vi "Bipolar Output (Read).vi"(6 "ISOBUS address":T2=-1 caption="ISOBUS address (-1)", 8 "error in":errorcluster, 11 "Mercury Reference In":T3) -> (0 "error out":errorcluster, 2 "Bipolar Output":string, 3 "Mercury Reference Out":T3, 4 "Valid?":T1)   [LabVIEW 2013, in "Mercury iXX.lvlib" / "Magnet.lvlib"]
doc: "Read the Bipolar output mode of the selected magnet PSU."
uses:
  <instrlib>/Mercury iXX/Public/Libraries/Magnet.lvlib
  <instrlib>/Mercury iXX/Public/Controls/Mercury Reference.ctl
  <instrlib>/Mercury iXX/Public/Controls/Comms Transport Layer.ctl
  <instrlib>/Mercury iXX/Private/Controls/Query Dynamic Reference.ctl
  <instrlib>/Mercury iXX/Public/Controls/ISOBus Address.ctl
  <instrlib>/Mercury iXX/Public/Controls/Is Valid LED.ctl
  <instrlib>/Mercury iXX/Private/Controls/Command Verbs.ctl
  <instrlib>/Mercury iXX/Mercury iXX.lvlib
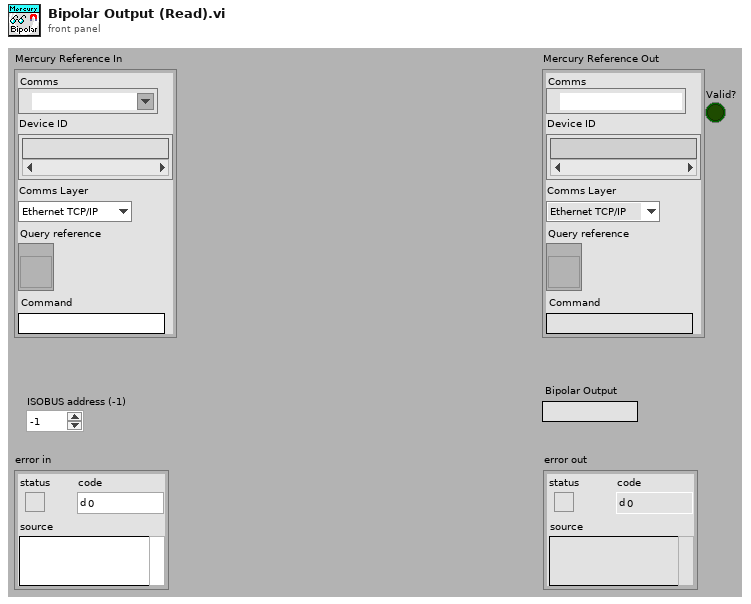
[diagram p1: front panel]
types:
  T1 = typedef "Mercury iXX.lvlib/Is Valid LED.ctl" = bool
  T2 = typedef "Mercury iXX.lvlib/ISOBus Address.ctl" = i32
  T3 = typedef "Mercury iXX.lvlib/Mercury Reference.ctl" = cluster{"Comms":refnum<visa-resource-name>, "Device ID":string[], "Comms Layer":T4, "Command":string, "Query reference":T5}
  T4 = typedef "Mercury iXX.lvlib/Comms Transport Layer.ctl" = enum16{"Ethernet TCP/IP", "USB", "ISOBus - RS-232", "GPIB"}
  T5 = typedef "Mercury iXX.lvlib/Query Dynamic Reference.ctl" = refnum<vi>
  T6 = typedef "Mercury iXX.lvlib/Command Verbs.ctl" = string
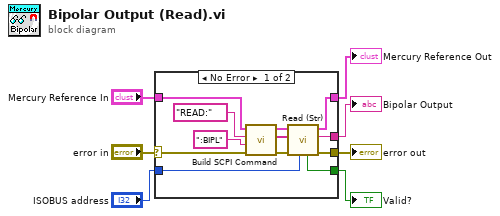
[diagram p0: block diagram]
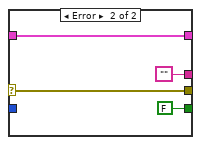
[diagram p2: hidden frame]
diagram:
  n1 = case shown="No Error" "error in" {
    selector: "error in" -> [w18 w22]
    tunnel: "Mercury Reference In" -> [w19 w23]
    tunnel: [w12 w23] -> w6
    tunnel: [w8 w22] -> w5
    tunnel: "ISOBUS address" -> [w10 _]
    tunnel: [w9 T1 FALSE ("Valid?")] -> w3
    tunnel: [w11 ""] -> w2
    frame No Error {
      n2 = call <instrlib>:"Build SCPI Command.vi"("error in"=w18, "Noun(s)"=":BIPL" ("Command"), "Verb"=T6 "READ:", "Mercury Reference In"=w19) -> ("error out"=w14:errorcluster, "SCPI Message(s)"=w13:string[], "Mercury Reference Out"=w15:T3)  [unwired: 5 out]
      n3 = call <instrlib>:"Read (Str).vi"("ISOBUS address"=w10, "error in"=w14, "SCPI Message(s)"=w13, "Mercury Reference In"=w15) -> ("error out"=w8:errorcluster, "Response"=w11:string, "Mercury Reference Out"=w12:T3, "Valid?"=w9:T1)  [unwired: 4 out]
    }
    frame Error {
    }
  }
  "Mercury Reference Out" <- w6
  "error out" <- w5
  "Valid?" <- w3
  "Bipolar Output" <- w2
